vi "SetExposure.vi"(8 "error in (no error)":errorcluster, 10 "Setting.Exposure":i32, 11 "Camera_Prime95B in":refnum<class "Camera_Prime95B.lvclass">) -> (0 "error out":errorcluster, 3 "Camera_Prime95B out":refnum<class "Camera_Prime95B.lvclass">)   [LabVIEW 2020, in "Camera_Prime95B.lvlib" / "Camera_Prime95B.lvclass"]
uses:
  Camera_Prime95B.lvclass
  Camera_Prime95B.lvclass/Camera_Prime95B.ctl
  E:/Development/DevHardSoftware/MicroscopyFramework/Model/Hardware Layer/Real Hardware/Camera_Prime95B/Camera_Prime95B/Dependencies/PVCamNET.dll
  Dependencies/PVCamNET.dll
  Controls/Wait For Stop Status.ctl
  Hardware Abstraction Layer/Component/Camera/Camera/Camera.lvclass
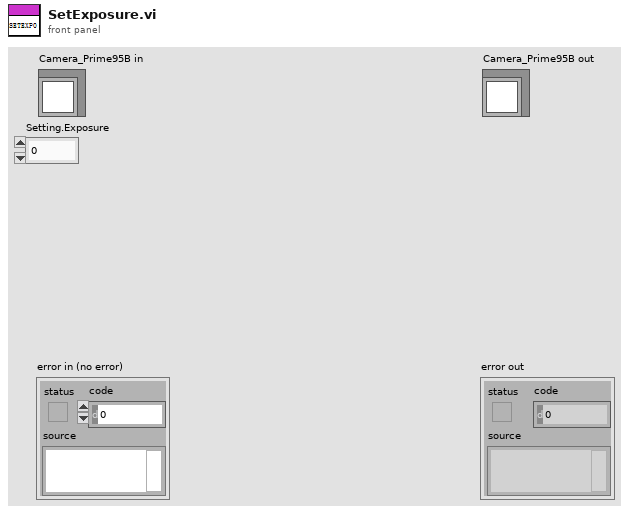
[diagram p1: front panel]
types:
  T1 = typedef "Device.lvlib/DeviceStatus.ctl" = i32
  T2 = typedef "Camera_Prime95B.lvlib/Camera_Prime95B.lvclass/Wait For Stop Status.ctl" = i32
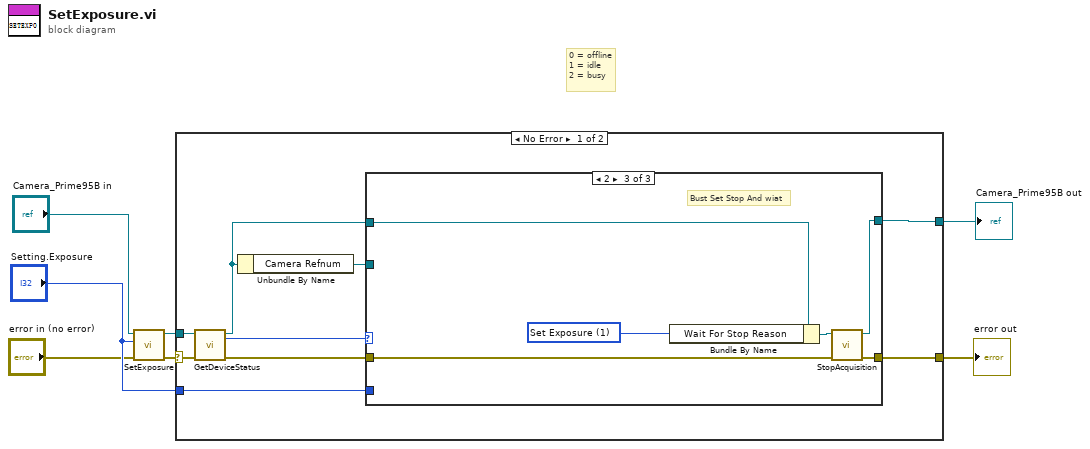
[diagram p0: block diagram]
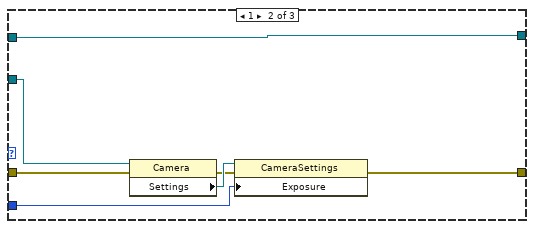
[diagram p3: hidden frame]
diagram:
  # "0 = offline\n1 = idle\n2 = busy"
  n1 = call-parent "SetExposure.vi"("error in (no error)"="error in (no error)", "Setting.Exposure"="Setting.Exposure", "Camera in"="Camera_Prime95B in") -> ("error out"=w3:errorcluster, "Camera out"=w4:refnum<class "Camera_Prime95B.lvclass">)  [unwired: 7 in]
  n2 = case shown="No Error" w3 {
    selector: w3 -> [w14 w33]
    tunnel: [w15 w33] -> w1
    tunnel: w4 -> [w13 w32]
    tunnel: "Setting.Exposure" -> [w16 _]
    tunnel: [w8 w32] -> w2
    frame No Error {
      n3 = call-dynamic "GetDeviceStatus.vi"("error in (no error)"=w14, "Camera_Prime95B in"=w13) -> ("error out"=w11:errorcluster, "Status"=w12:T1, "Camera_Prime95B out"=w9:refnum<class "Camera_Prime95B.lvclass">)  [unwired: 7 in]
      n4 = Unbundle By Name(w9) -> ("Camera Refnum"=w10:refnum<k24>)
      n5 = case shown="2" w12 {
        tunnel: [w18 w25 w30] -> w15
        tunnel: w10 -> [_ w22 _]
        tunnel: w16 -> [_ w21 _]
        tunnel: w11 -> [w18 w20 w31]
        tunnel: w9 -> [w17 w19 w27]
        tunnel: [w17 w19 w28] -> w8
        frame 0, Default {
        }
        frame 1 {
          n6 = property class="Camera"(reference=w22, error in=w20) -> (error out=w23:errorcluster, "Settings"=w24:refnum<k24>)  [unwired: 1 out]
          n7 = property class="CameraSettings"(reference=w24, error in=w23, "Exposure"=w21) -> (error out=w25:errorcluster)  [unwired: 1 out]
        }
        frame 2 {
          w29 = T2 1 items=["None", "Set Exposure", "Set Binning", "Set ROI", "Senquen Acq", ""] ("Wait For Stop Reason")
          # "Bust Set Stop And wiat"
          n8 = Bundle By Name(cluster=w27, "Wait For Stop Reason"=w29) -> (w26:refnum<class "Camera_Prime95B.lvclass">)
          n9 = call-dynamic "StopAcquisition.vi"("error in (no error)"=w31, "Camera_Prime95B in"=w26) -> ("error out"=w30:errorcluster, "Camera_Prime95B out"=w28:refnum<class "Camera_Prime95B.lvclass">)  [unwired: 8 in]
        }
      }
    }
    frame Error {
    }
  }
  "error out" <- w1
  "Camera_Prime95B out" <- w2
